vi "Random Number Assert.vi"   [LabVIEW 2016]
uses:
  Core/AssertEngine/AssertEngine.lvlib
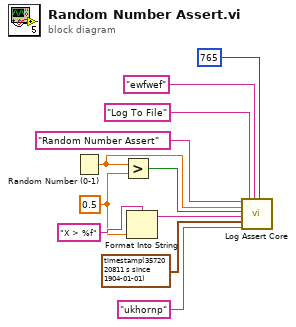
[diagram p0: block diagram]
diagram:
  w6 = 0.5 ("y")
  n1 = Random Number (0-1)() -> (number: 0 to 1=w9:dbl)
  n2 = Greater?(x=w9, y=w6) -> (0:w8:bool)
  n3 = Format Into String(format string="X > %f", w6) -> (resulting string=w5:string)  [unwired: 2 in, 1 out]
  n4 = call "Log Assert Core.vi"("Assert Name"="Random Number Assert", "Data Value"=w9, "Passed?"=w8, "Eval String"=w5, "Build Timestamp"=timestamp(3572020811.1610465 s since 1904-01-01) ("Time Stamp"), "Assert Builder"="ukhornp", "Default Failure Action"="Log To File", "Comment"="ewfwef", "Assert VI UID"=765) -> ()  [unwired: 11 in]
